vi "GEA2 Script_Parse Flags.vi"(0 "Flag String":string, 5 "Default wait time (s)":dbl, 7 "Default Continue if stopped?":bool, 11 "Error In":errorcluster) -> (4 "Wait time (s)":dbl, 6 "Continue if stopped?":bool, 15 "Error Out":errorcluster)   [LabVIEW 2014]
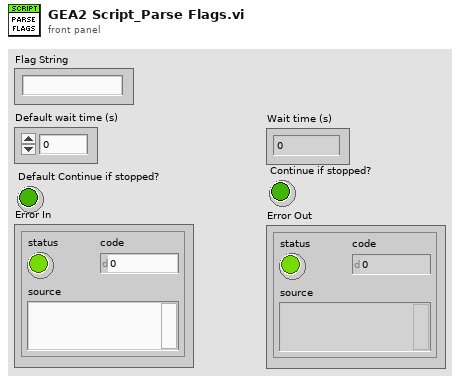
[diagram p1: front panel]
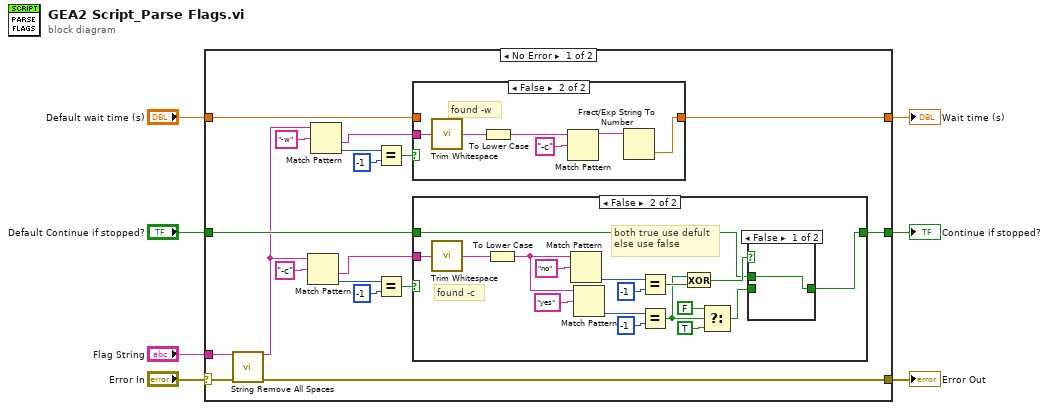
[diagram p0: block diagram]
diagram:
  n1 = case shown="No Error" "Error In" {
    selector: "Error In" -> [w9 w55]
    tunnel: [w8 w55] -> w6
    tunnel: "Flag String" -> [w16 _]
    tunnel: [w23 w54] -> w4
    tunnel: "Default Continue if stopped?" -> [w22 w54]
    tunnel: "Default wait time (s)" -> [w11 w53]
    tunnel: [w10 w53] -> w1
    frame No Error {
      n2 = call "String Remove All Spaces.vi"("Input String"=w16, "error in (no error)"=w9) -> ("Spaces Removed"=w15:string, "error out"=w8:errorcluster)  [unwired: 12 in]
      n3 = Match Pattern(string=w15, regular expression="-c") -> (after substring=w18:string, offset past match=w21:i32)  [unwired: 1 in, 2 out]
      n4 = Match Pattern(string=w15, regular expression="-w") -> (after substring=w17:string, offset past match=w12:i32)  [unwired: 1 in, 2 out]
      n5 = Equal?(x=w12, y=-1) -> (x = y?=w13:bool)
      n6 = Equal?(x=w21, y=-1) -> (x = y?=w19:bool)
      n7 = case shown="False" w13 {
        tunnel: w17 -> [_ w32]
        tunnel: [w26 w27] -> w10
        tunnel: w11 -> [w26 _]
        frame True {
          # "did not find -w\nuse default"
        }
        frame False {
          # "found -w"
          n8 = call <vilib>:"Trim Whitespace.vi"("string"=w32) -> ("trimmed string"=w31:string)  [unwired: 1 in]
          n9 = To Lower Case(string=w31) -> (all lower case string=w29:string)
          n10 = Match Pattern(string=w29, regular expression="-c") -> (before substring=w28:string)  [unwired: 1 in, 3 out]
          n11 = Fract/Exp String To Number(string=w28) -> (number=w27:dbl)  [unwired: 3 in, 1 out]
        }
      }
      n12 = case shown="False" w19 {
        tunnel: [w33 w38] -> w23
        tunnel: w22 -> [w33 w39]
        tunnel: w18 -> [_ w50]
        frame True {
          # "did not find -c\nuse default"
        }
        frame False {
          # "both true use defult\nelse use false"
          # "found -c"
          n13 = call <vilib>:"Trim Whitespace.vi"("string"=w50) -> ("trimmed string"=w49:string)  [unwired: 1 in]
          n14 = To Lower Case(string=w49) -> (all lower case string=w42:string)
          n15 = Match Pattern(string=w42, regular expression="no") -> (offset past match=w45:i32)  [unwired: 1 in, 3 out]
          n16 = Match Pattern(string=w42, regular expression="yes") -> (offset past match=w46:i32)  [unwired: 1 in, 3 out]
          n17 = Equal?(x=w45, y=-1) -> (x = y?=w41:bool)
          n18 = Equal?(x=w46, y=-1) -> (x = y?=w37:bool)
          n19 = Exclusive Or(1:w41, 2:w37) -> (0:w40:bool)
          n20 = Select(t=FALSE, s=w37, f=TRUE) -> (s? t:f=w34:bool)
          n21 = case shown="False" w40 {
            tunnel: w39 -> [w51 _]
            tunnel: [w51 w52] -> w38
            tunnel: w34 -> [_ w52]
            frame False {
            }
            frame True {
            }
          }
        }
      }
    }
    frame Error {
    }
  }
  "Error Out" <- w6
  "Continue if stopped?" <- w4
  "Wait time (s)" <- w1
